vi "I2C Read.vi"(1 "Min time SCl low (uSec)":u32, 2 "Min Time SCL high (uSec)":u32, 4 "Number of Bytes":i16) -> (0 "Data bit array":bool[](array[boolean]))   [LabVIEW 2013]
uses:
  <vilib>/rvi/Emulation/niFpgaSctlEmulationGetInTimedLoop.vi
  <vilib>/rvi/Emulation/niFpgaEmulationReportErrorSimple.vi
  <vilib>/rvi/Emulation/niFpgaGetClockAttributes.vi
  <vilib>/rvi/eio/common/nirviEmuTemplateMethod_errors.vi
  <vilib>/rvi/Emulation/niFpgaCriticalErrorInLSC.vi
  <vilib>/eio/EIONode/EIONode.xnode
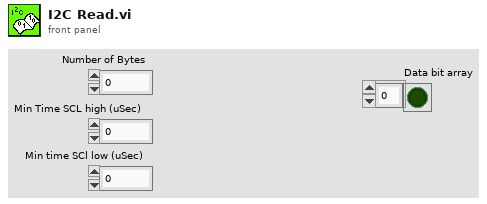
[diagram p1: front panel]
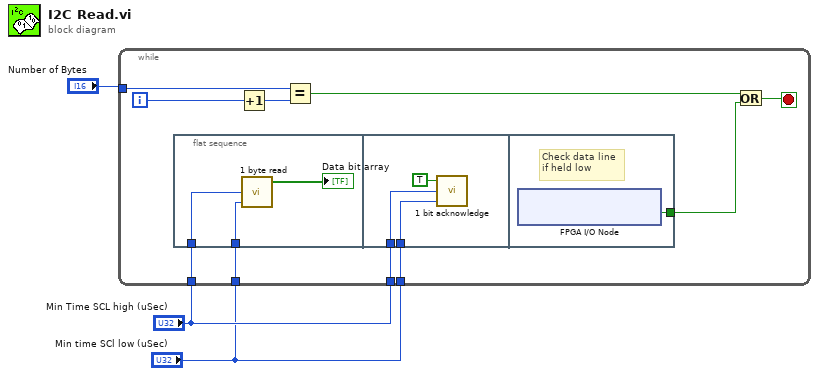
[diagram p0: block diagram]
diagram:
  n1 = while {
    tunnel: "Number of Bytes" -> [w11]
    tunnel: "Min Time SCL high (uSec)" -> [w10]
    tunnel: "Min time SCl low (uSec)" -> [w9]
    tunnel: "Min Time SCL high (uSec)" -> [w8]
    tunnel: "Min time SCl low (uSec)" -> [w7]
    i -> [w12]
    stop <- w6 stop-if-true
    n2 = flat-sequence {
      tunnel: w10 -> [w16]
      tunnel: w9 -> [w15]
      tunnel: w8 -> [w18]
      tunnel: w7 -> [w17]
      tunnel: [w20] -> w4
      frame #0 {
        n3 = call "1 byte read.vi"("Min time SCL low (uSec)"=w15, "Min Time SCL high (uSec)"=w16) -> ("Data bit array"=→"Data bit array":bool[])  [unwired: 3 in]
      }
      frame #1 {
        n4 = call "1 bit acknowledge.vi"("Min time SCL low (uSec)"=w17, "Min Time SCL high (uSec)"=w18, "Acknowledgement"=TRUE) -> ()  [unwired: 1 in]
      }
      frame #2 {
        # "Check data line\nif held low"
        n5 = xnode "FPGA I/O Node"() -> ("ConnectorB/DIO13"=w20:bool)  [unwired: 1 in, 1 out]
      }
    }
    n6 = Increment(x=w12) -> (x+1=w13:i32)
    n7 = Equal?(x=w11, y=w13) -> (x = y?=w5:bool)
    n8 = Or(x=w5, y=w4) -> (x .or. y?=w6:bool)
  }
